vi "DAQmx Timing (Burst Import Clock).vi"(0 "task/channels in":refnum<k21>, 1 "sample mode":i32(ring)=10178 items=["Finite Samples"=10178, "Continuous Samples"=10123, "Hardware Timed Single Point"=12522], 2 "samples per channel":i32=1000, 5 "sample clock rate":dbl=1000.0, 7 "sample clock source":tag, 9 "sample clock active edge":i32(ring)=10280 items=["Rising"=10280, "Falling"=10171], 11 "error in":errorcluster, 12 "pause when":i32(ring)=10192 items=["High"=10192, "Low"=10214], 13 "ready for transfer event active level":i32(ring)=10095 items=["Active High"=10095, "Active Low"=10096]) -> (4 "task out":refnum<k21>, 15 "error out":errorcluster)   [LabVIEW 2020]
doc: "Configures when the DAQ device transfers data to a peripheral device, using an imported sample clock to control burst handshake timing."
uses:
  nilvaiu.dll
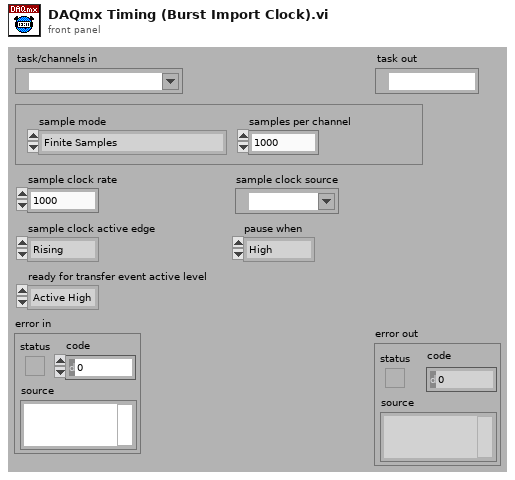
[diagram p1: front panel]
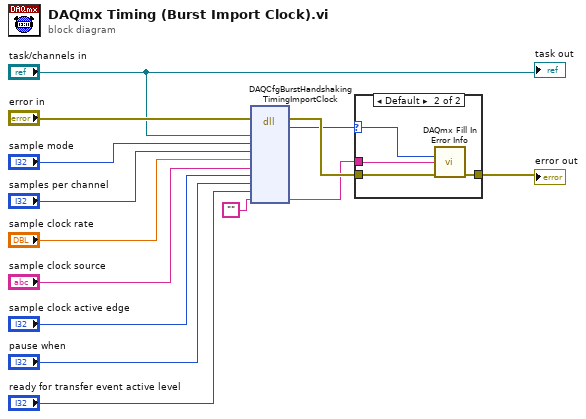
[diagram p0: block diagram]
diagram:
  n1 = dll-call lib="nilvaiu.*" fn="DAQCfgBurstHandshakingTimingImportClock"(error in="error in", "taskID"="task/channels in", "sampleMode"="sample mode", "samplesPerChannel"="samples per channel", "rate"="sample clock rate", "source"="sample clock source", "activeEdge"="sample clock active edge", "pauseWhen"="pause when", "readyForTransferEventActiveLevel"="ready for transfer event active level", "extendedErrorInfo"="") -> (error out=w11:errorcluster, "return type"=w9:i32, "extendedErrorInfo"=w10:string)  [unwired: 4 in, 7 out]
  n2 = case shown="Default" w9 {
    selector: w9 -> [_ w17]
    tunnel: w11 -> [w15 w19]
    tunnel: [w15 w18] -> w13
    tunnel: w10 -> [_ w16]
    frame 0 {
    }
    frame Default {
      n3 = call "DAQmx Fill In Error Info.vi"("status code"=w17, "extended error info"=w16, "error in"=w19) -> ("error out"=w18:errorcluster)  [unwired: 1 in, 11 out]
    }
  }
  "error out" <- w13
  "task out" <- "task/channels in"
